vi "Generate Simulated Data.vi"(7 "Type de mode":bool, 8 "error in (no error)":T2 caption="entrée d'erreur (pas d'erreur)", 9 "Péri":tag="Dev1", 10 "Longueur d'onde":dbl, 11 "Type de signal":T1) -> (0 "error out":T2 caption="sortie d'erreur", 2 "Données du graphe":waveform(dbl)[](array[waveform]))   [LabVIEW 2018, in "Acquisition.lvlib"]
doc: "Génère des exemples de waveforms en fonction du type de signal dans l'entrée Configuration du matériel."
uses:
  Acquisition.lvlib
  Signal Type.ctl
  <vilib>/Analysis/baseanly.llb/Mean (DBL).vi
  <vilib>/Analysis/NI_AALBase.lvlib
panel:
  out "Graphe déroulant":dynamicdata(graph)
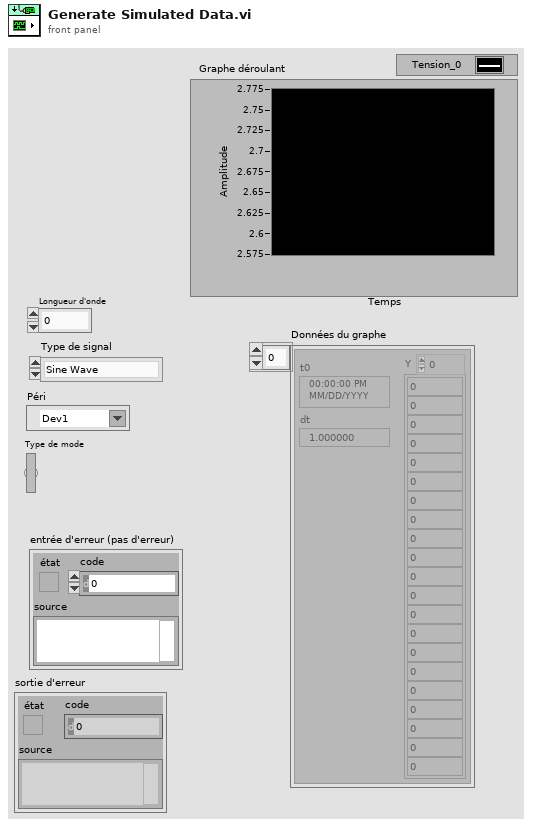
[diagram p1: front panel]
types:
  T1 = typedef "Acquisition.lvlib/Signal Type.ctl" = enum16{"Sine Wave", "Square with Noise", "Signal triangulaire", "Simulation DAQ"}
  T2 = cluster{"état":bool, "code":i32, "source":string}
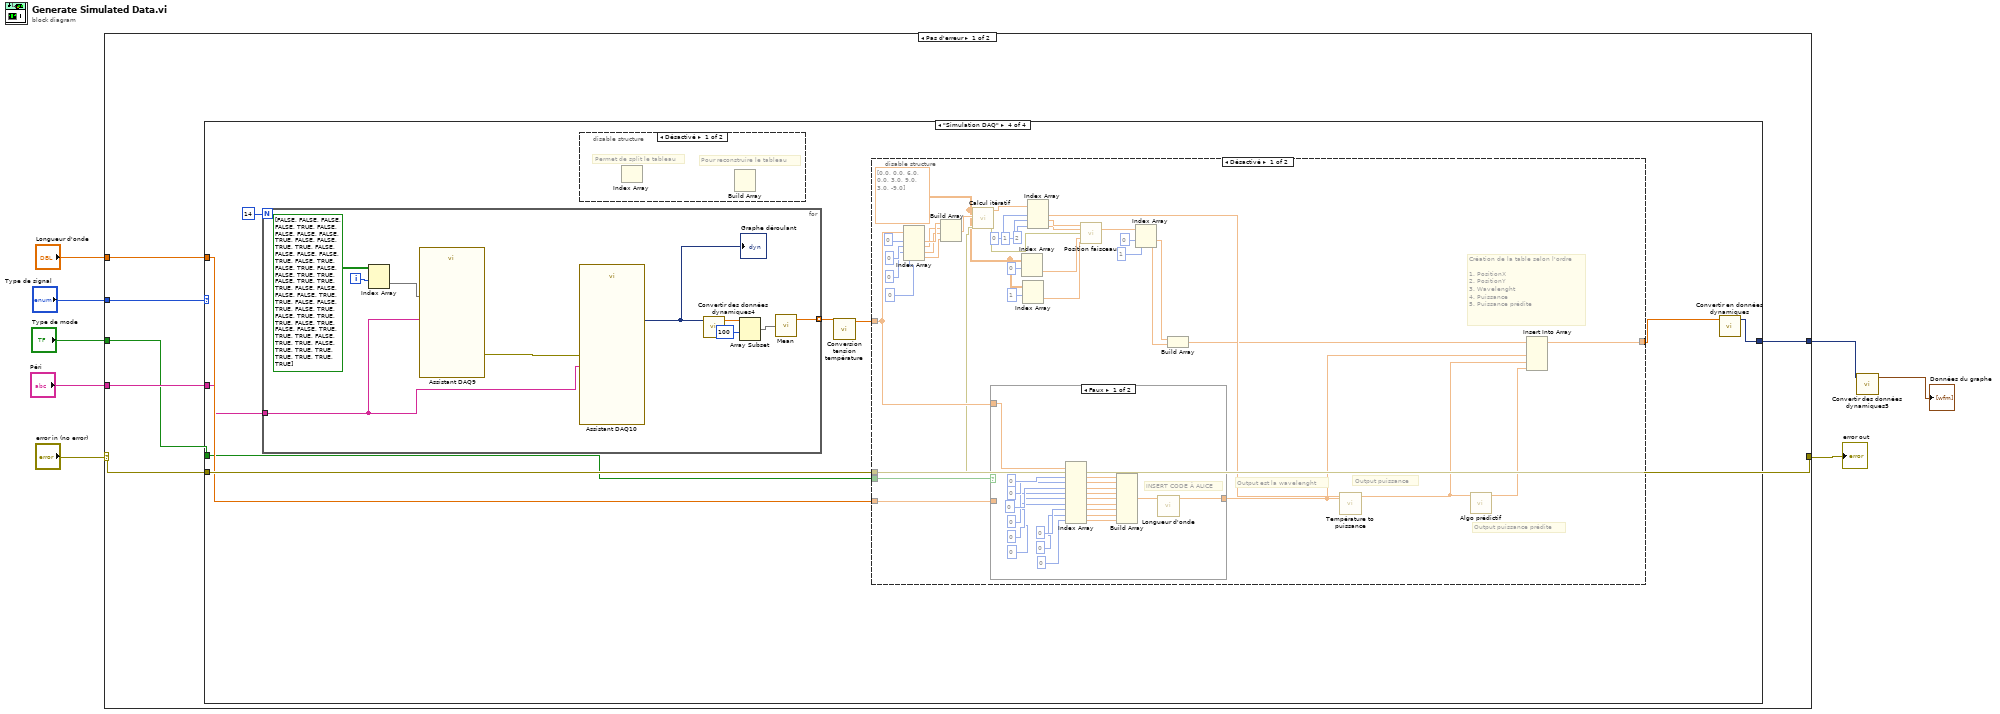
[diagram p0: block diagram]
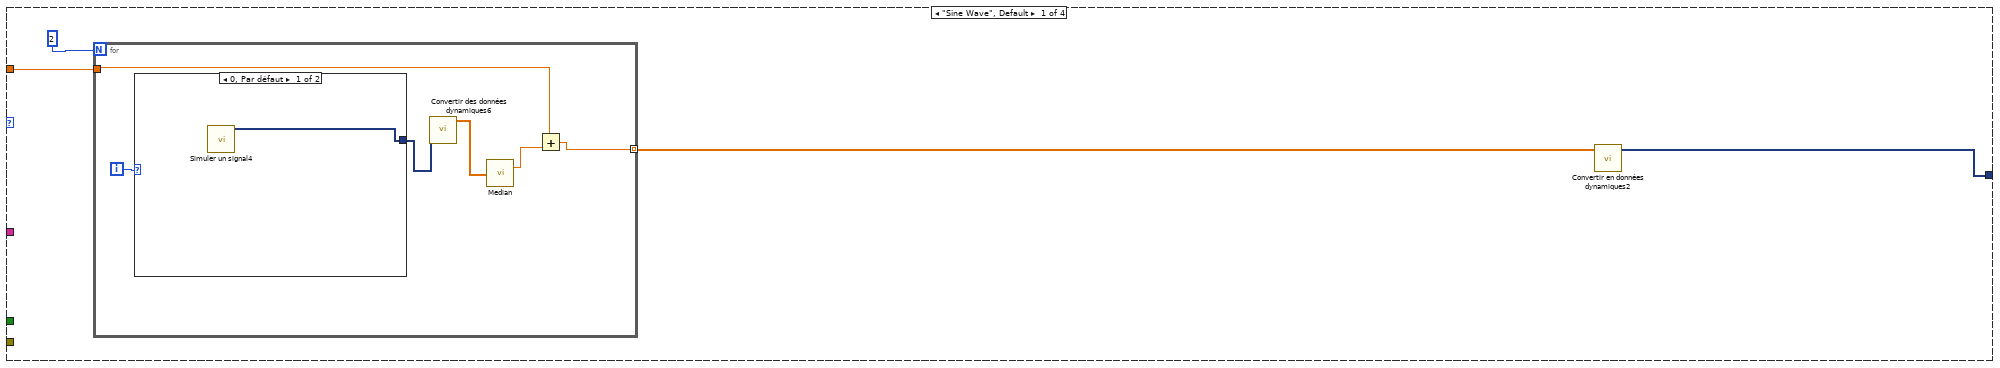
[diagram p2: hidden frame]
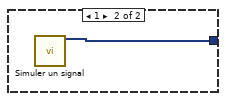
[diagram p3: hidden frame]
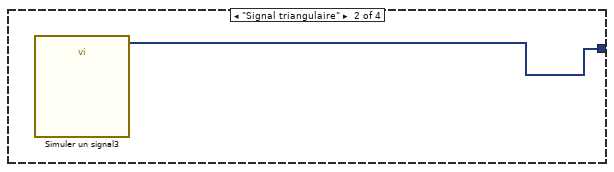
[diagram p4: hidden frame]
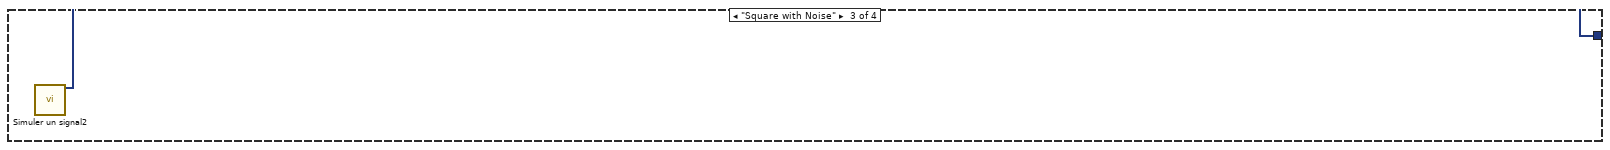
[diagram p5: hidden frame]
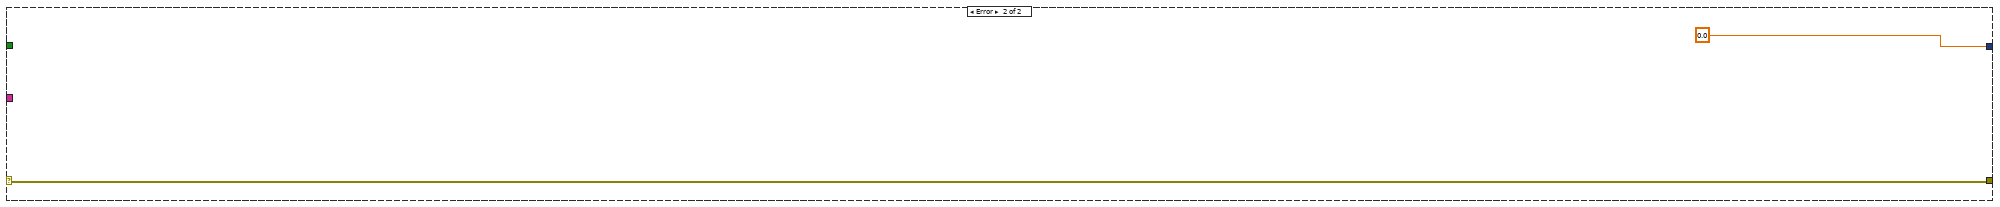
[diagram p9: hidden frame]
diagram:
  n1 = case shown="Pas d'erreur" "error in (no error)" {
    selector: "error in (no error)" -> [w9 w108]
    tunnel: [w9 w108] -> w7
    tunnel: "Type de signal" -> [w14 _]
    tunnel: [w13 0.0] -> w4
    tunnel: "Longueur d'onde" -> [w12 _]
    tunnel: "Péri" -> [w11 _]
    tunnel: "Type de mode" -> [w10 _]
    frame No Error {
      n2 = case shown="\"Simulation DAQ\"" w14 {
        tunnel: [w17 w27 w28 w36] -> w13
        tunnel: w12 -> [w16 _ _ w35]
        tunnel: w11 -> [_ _ _ w34]
        tunnel: w10 -> [_ _ _ w33]
        tunnel: w9 -> [_ _ _ w29]
        frame "Sine Wave", Default {
          n3 = for {
            N: 2 -> [_]
            tunnel: [w20] -> w15 mode=indexing
            tunnel: w16 -> [w19]
            i -> [w24]
            n4 = case shown="0, Par défaut" w24 {
              tunnel: [w25 w26] -> w23
              frame 0, Default {
                n5 = call "Simuler un signal4"() -> ("CC"=w25:dynamicdata)  [unwired: 14 in, 1 out]
              }
              frame 1 {
                n6 = call "Simuler un signal"() -> ("Sinus avec Bruit uniforme"=w26:dynamicdata)  [unwired: 14 in, 1 out]
              }
            }
            n7 = call "Convertir des données dynamiques6"("Dynamic Data Type"=w23) -> ("Array"=w22:dbl[])  [unwired: 3 in]
            n8 = call <vilib>:"Median.vi"("X"=w22) -> ("median"=w21:dbl)  [unwired: 1 out]
            n9 = Add(x=w19, y=w21) -> (x+y=w20:dbl)
          }
          n10 = call "Convertir en données dynamiques2"("Array"=w15) -> ("Dynamic Data Type"=w17:dynamicdata)  [unwired: 3 in]
        }
        frame "Signal triangulaire" {
          n11 = call "Simuler un signal3"() -> ("Triangle"=w27:dynamicdata)  [unwired: 14 in, 1 out]
        }
        frame "Square with Noise" {
          n12 = call "Simuler un signal2"() -> ("Square with Gaussian Noise"=w28:dynamicdata)  [unwired: 14 in, 1 out]
        }
        frame "Simulation DAQ" {
          n13 = for {
            N: 14 -> [_]
            tunnel: [w98] -> w31 mode=indexing
            tunnel: w34 -> [w97]
            i -> [w104]
            n14 = Index Array(array=bool[][] [[FALSE, FALSE, FALSE, FALSE], [TRUE, FALSE, FALSE, FALSE], [FALSE, TRUE, FALSE, FALSE], [TRUE, TRUE, FALSE, FALSE], [FALSE, FALSE, TRUE, FALSE], [TRUE, FALSE, TRUE, FALSE], [FALSE, TRUE, TRUE, FALSE], [TRUE, TRUE, TRUE, FALSE], [FALSE, FALSE, FALSE, TRUE], [TRUE, FALSE, FALSE, TRUE], [FALSE, TRUE, FALSE, TRUE], [TRUE, TRUE, FALSE, TRUE], [FALSE, FALSE, TRUE, TRUE], [TRUE, FALSE, TRUE, TRUE], [FALSE, TRUE, TRUE, TRUE], [TRUE, TRUE, TRUE, TRUE]], index (row)=w104) -> (element=w103:bool[])  [unwired: 1 in]
            n15 = call "Assistant DAQ9"("data"=w103, "nom du périphérique"=w97) -> ("error out"=w106:errorcluster)  [unwired: 16 in, 1 out]
            n16 = call "Assistant DAQ10"("error in"=w106, "nom du périphérique"=w97) -> ("data"=w102:dynamicdata)  [unwired: 15 in, 2 out]
            "Graphe déroulant" <- w102
            n17 = call "Convertir des données dynamiques4"("Dynamic Data Type"=w102) -> ("Array"=w101:dbl[])  [unwired: 3 in]
            n18 = Array Subset(array=w101, index=100 ("indice")) -> (w99:dbl[])  [unwired: 1 in]
            n19 = call-poly <vilib>:"Mean.vi"("X"=w99) -> ("mean"=w98:dbl)  [unwired: 1 out]
          }
          n20 = disable-structure shown="Désactivé" {
            frame Disabled {
              # "Pour reconstruire le tableau"
              # "Permet de split le tableau"
              n21 = Index Array() -> ()  [unwired: 2 in, 1 out]
              n22 = Build Array() -> ()  [unwired: 4 in, 1 out]
            }
            frame Enabled {
            }
          }
          n23 = call "Conversion tension température.vi"("Tension In"=w31) -> ("Température Out"=w30:dbl[])  [unwired: 10 in]
          n24 = disable-structure shown="Désactivé" {
            disable-tunnel: w35 -> [w73 _]
            disable-tunnel: w33 -> [w72 _]
            disable-tunnel: [w71 w96] -> w32
            disable-tunnel: w30 -> [w70 w96]
            disable-tunnel: w29 -> [w69 _]
            frame Disabled {
              w65 = dbl[][] [[0.0, 0.0], [6.0, 0.0], [3.0, 9.0], [3.0, -9.0]] ("Position des capteurs")
              # "Output puissance prédite"
              # "Création de la table selon l'ordre\n\n1. PositionX\n2. PositionY\n3. Wavelenght\n4. Puissance\n5. Puissance prédite"
              # "Output puissance"
              # "Output est la wavelenght"
              n25 = Index Array(array=w70, index #1=0, index #2=0, index #3=0, index #4=0) -> (element #1=w67:dbl, element #2=w52:dbl, element #3=w51:dbl, element #4=w50:dbl)
              n26 = Build Array(w67, w52, w51, w50) -> (w68:dbl[])
              n27 = call "Calcul itératif.vi"("error in (no error)"=w69, "Température capteur 1-2-3-4-Ambiant"=w68, "Position des capteurs"=w65) -> ("error out"=w38:T2, "DATA - T/R1/R2/R3"=w46:dbl[])  [unwired: 7 in]
              n28 = case shown="Faux" w72 {
                tunnel: [w83 w95] -> w41
                tunnel: w73 -> [_ w95]
                tunnel: w70 -> [w94 _]
                frame False {
                  # "INSERT CODE À ALICE"
                  n29 = Index Array(array=w94, index #1=0 ("indice"), index #2=0 ("indice"), index #3=0 ("indice"), index #4=0 ("indice"), index #5=0 ("indice"), index #6=0 ("indice"), index #7=0 ("indice"), index #8=0 ("indice"), index #9=0 ("indice")) -> (element #1=w82:dbl, element #2=w81:dbl, element #3=w80:dbl, element #4=w79:dbl, element #5=w78:dbl, element #6=w77:dbl, element #7=w76:dbl, element #8=w75:dbl, element #9=w74:dbl)
                  n30 = Build Array(w82, w81, w80, w79, w78, w77, w76, w75, w74) -> (w93:dbl[])
                  n31 = call "Longueur d'onde.vi"("T thermistances"=w93) -> ("Longeur d'onde"=w83:dbl)  [unwired: 10 in]
                }
                frame True {
                }
              }
              n32 = Index Array(array=w65, index (row)=0 ("indice (ligne)")) -> (element=w64:dbl[])  [unwired: 1 in]
              n33 = Index Array(array=w65, index (row)=1 ("indice (ligne)")) -> (element=w63:dbl[])  [unwired: 1 in]
              n34 = Index Array(array=w46, index #1=0, index #2=1 ("indice"), index #3=2 ("indice")) -> (element #1=w43:dbl, element #2=w45:dbl, element #3=w44:dbl)
              n35 = call "Position faisceau.vi"("R1"=w45, "R2"=w44, "error in (no error)"=w38, "Capteur 1"=w64, "Capteur 2"=w63) -> ("Coord"=w60:dbl[])  [unwired: 9 in, 1 out]
              n36 = Index Array(array=w60, index #1=0 ("indice"), index #2=1 ("indice")) -> (element #1=w57:dbl, element #2=w56:dbl)
              n37 = Build Array(w57, w56) -> (w42:dbl[])
              n38 = call "Température to puissance.vi"("Longueur d'onde"=w41, "Température max"=w43) -> ("Puissance"=w39:dbl)  [unwired: 9 in]
              n39 = call "Algo prédictif.vi"("Puissance intan."=w39) -> ("Puissance prédite"=w40:dbl)  [unwired: 10 in]
              n40 = Insert Into Array(array=w42, new element #1=w41, new element #2=w39, new element #3=w40) -> (w71:dbl[])  [unwired: 1 in]
            }
            frame Enabled {
            }
          }
          n41 = call "Convertir en données dynamiques"("Array"=w32) -> ("Dynamic Data Type"=w36:dynamicdata)  [unwired: 3 in]
        }
      }
    }
    frame Error {
    }
  }
  "error out" <- w7
  n42 = call "Convertir des données dynamiques5"("Dynamic Data Type"=w4) -> ("Array of Waveform"=→"Données du graphe":waveform(dbl)[])  [unwired: 3 in]
